vi "UDP__ReceiveDataViaSystemEvent.vi"(6 "Event Registration Ref IN":T1, 8 "error in":errorcluster, 11 "Timeout":i32=5000) -> (0 "error out":errorcluster, 2 "Parameters":string[](array[string]), 3 "Command":string, 4 "Event Registration Ref OUT":T1)   [LabVIEW 2022 SP3, in "hse-network.lvlib"]
doc: "____\nHAMPEL SOFTWARE ENGINEERING v3.8.0 (2023-12-18 14:41)"
uses:
  hse-network.lvlib
  hse-misc/Event/Event_GenericRegistration.ctl
  hse-misc/Event/Event_GenericReference.ctl
  hse-misc/Event/Event_GenericDatatype.ctl
  hse-misc/hse-misc.lvlib
panel:
  out "Event Parameter":string
  out "Event Name":string
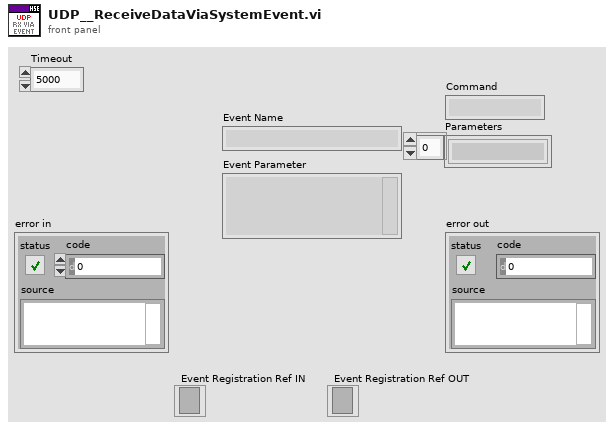
[diagram p1: front panel]
types:
  T1 = typedef "hse-misc.lvlib/Event_GenericRegistration.ctl" = refnum<event-registration>
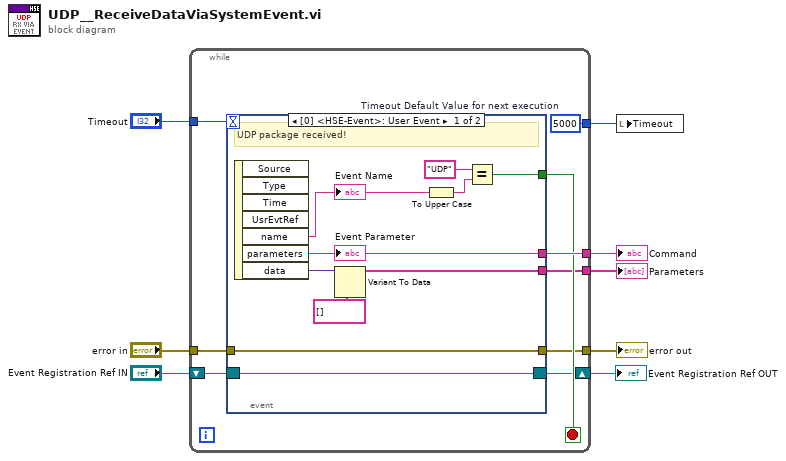
[diagram p0: block diagram]
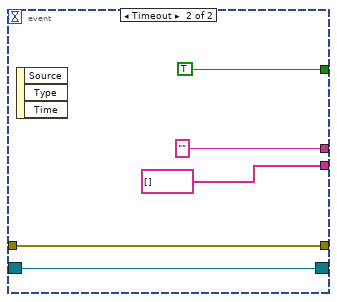
[diagram p2: hidden frame]
diagram:
  n1 = while {
    tunnel: "error in" -> [w17]
    tunnel: [w13] -> w8
    tunnel: [w16] -> w7
    shift-right: [w14] -> w1
    shift-left: "Event Registration Ref IN" -> [w9]
    tunnel: "Timeout" -> [w12]
    tunnel: [w11] -> w4
    tunnel: [w10] -> w3
    stop <- w15 stop-if-true
    w11 = 5000  # Timeout Default Value for next execution
    n2 = event shown="[0] <HSE-Event>: User Event" {
      selector: w9 -> [w27 w29]
      dyn-events: [w27 w29] -> w14
      timeout: w12 -> [_ _]
      tunnel: [w21 "" ("Parameter")] -> w16
      tunnel: [w26 w30] -> w13
      tunnel: w17 -> [w26 w30]
      tunnel: [w23 TRUE] -> w15
      tunnel: [w18 string[] []] -> w10
      event User Event {
        # "UDP package received!"
        n3 = event-data() -> ("name"=w25:string, "parameters"=w21:string, "data"=w20:variant)  [unwired: 1 in, 4 out]
        "Event Name" <- w25
        "Event Parameter" <- w21
        n4 = Variant To Data(type=string[] [], Variant=w20) -> (data=w18:string[])  [unwired: 1 in, 1 out]
        n5 = To Upper Case(1:w25) -> (0:w22:string)
        n6 = Equal?(x="UDP", y=w22) -> (x = y?=w23:bool)
      }
      event Timeout {
        n7 = event-data() -> ()  [unwired: 1 in, 3 out]
      }
    }
  }
  "error out" <- w8
  "Command" <- w7
  "Parameters" <- w3
  "Event Registration Ref OUT" <- w1
  n8 = local write "Timeout"(w4) -> ()
